vi "Get Tree Data for Affected Item.vi"(7 "Action":T2, 10 "User VI Ref":refnum<vi>, 11 "Affected Items":T3) -> (2 "Use Dialog?":bool, 3 "Elements Array":T1[](array[typedef]))   [LabVIEW 2023]
doc: "Given one of the affected items, return the associated cluster type of that item.\n\nIf action is Rearrange or Delete, this will be an array of strings of the unble or unbundle by name terminals."
uses:
  top/BundleMagic.ctl
  controls/action enum.ctl
  cluster/Cluster Element Description.ctl
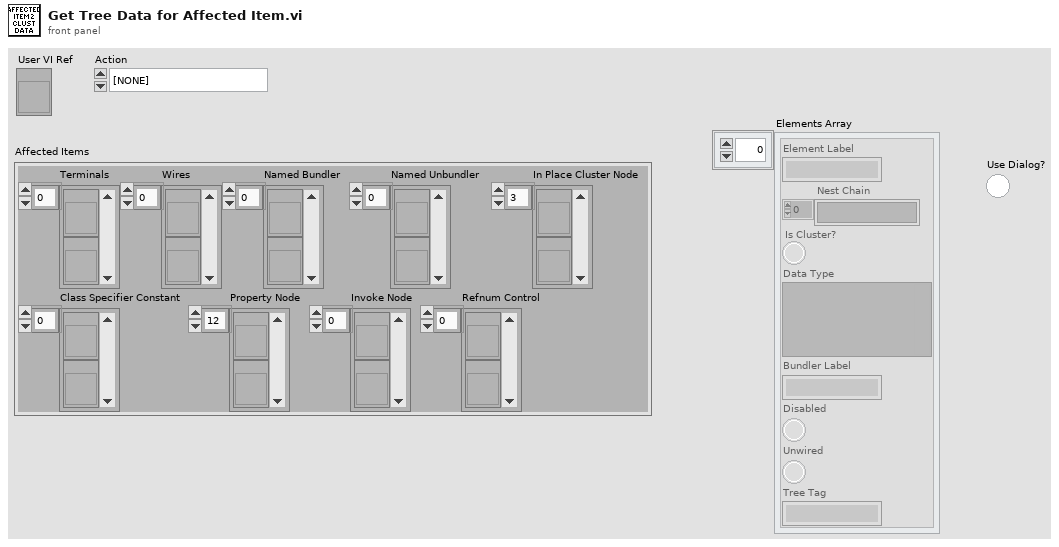
[diagram p1: front panel]
types:
  T1 = typedef "Cluster Element Description.ctl" = cluster{"Element Label":string, "Nest Chain":string[], "Is Cluster?":bool, "Data Type":variant, "Bundler Label":string, "Disabled":bool, "Unwired":bool, "Tree Tag":string}
  T2 = typedef "action enum.ctl" = enum16{"[NONE]", "Wire Bundle", "Wire Unbundle", "Terminal Unbundle", "Terminal Bundle", "Bundler Move Up", "Bundler Move Down", "Bundler Insert", "Bundler Remove", "Bundler Remove Unwired", "Bundler Rearrange", "In Place Insert", "In Place Remove", "In Place Remove Unwired", "In Place Rearrange", "Wire Properties", "Wire Method", "Terminal Properties", "Terminal Method", "Property Move Up", "Property Move Down", "Properties Insert", "Properties Remove", "Properties Remove Unwired", "Properties Rearrange", "Method Change", "Class for Constant", "Class For Control", "Class For Node", "Class Name to Clipboard"}
  T3 = typedef "BundleMagic.ctl" = cluster{"Terminals":refnum<vi>[], "Wires":refnum<vi>[], "Named Bundler":refnum<vi>[], "Named Unbundler":refnum<vi>[], "In Place Cluster Node":refnum<vi>[], "Class Specifier Constant":refnum<vi>[], "Property Node":refnum<vi>[], "Invoke Node":refnum<vi>[], "Refnum Control":refnum<vi>[]}
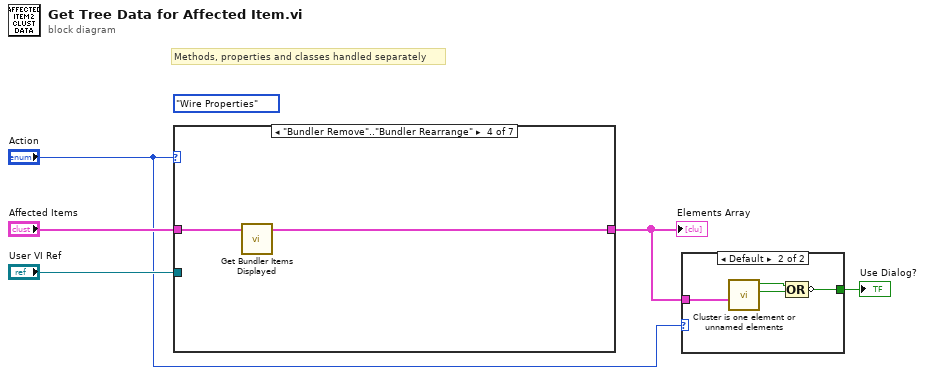
[diagram p0: block diagram]
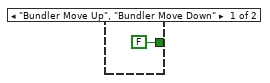
[diagram p2: hidden frame]
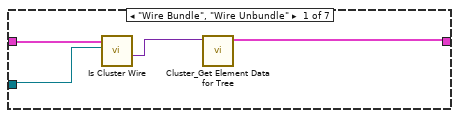
[diagram p3: hidden frame]
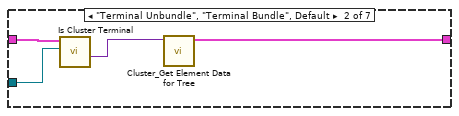
[diagram p4: hidden frame]
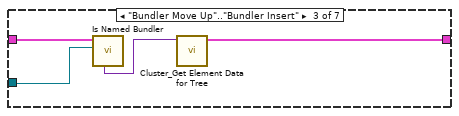
[diagram p5: hidden frame]
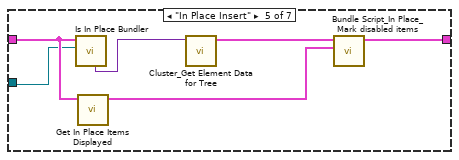
[diagram p6: hidden frame]
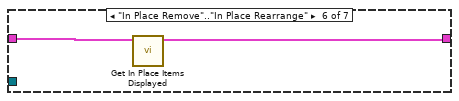
[diagram p7: hidden frame]
diagram:
  (unwired) action_enum."Wire Properties" ("Action")
  # "Methods, properties and classes handled separately"
  n1 = case shown="\"Bundler Remove\"..\"Bundler Rearrange\"" "Action" {
    tunnel: "Affected Items" -> [w9 w13 w17 w19 w24 w27 _]
    tunnel: "User VI Ref" -> [w8 w12 w16 _ w22 _ _]
    tunnel: [w6 w10 w14 w18 w23 w26 _] -> w2
    frame "Wire Bundle", "Wire Unbundle" {
      n2 = call "Is Cluster Wire.vi"("User VI Ref"=w8, "Affected Items"=w9) -> ("Data Type"=w7:variant)  [unwired: 6 in, 3 out]
      n3 = call "Cluster_Get Element Data for Tree.vi"("Data Type"=w7) -> ("Cluster Element Data Aray"=w6:T1[])  [unwired: 10 in]
    }
    frame "Terminal Unbundle", "Terminal Bundle", Default {
      n4 = call "Is Cluster Terminal.vi"("User VI Ref"=w12, "Affected Items"=w13) -> ("Data Type"=w11:variant)  [unwired: 7 in, 2 out]
      n5 = call "Cluster_Get Element Data for Tree.vi"("Data Type"=w11) -> ("Cluster Element Data Aray"=w10:T1[])  [unwired: 10 in]
    }
    frame "Bundler Move Up".."Bundler Insert" {
      n6 = call "Is Named Bundler.vi"("User VI Ref"=w16, "Affected Items"=w17) -> ("Data Type"=w15:variant)  [unwired: 3 in, 6 out]
      n7 = call "Cluster_Get Element Data for Tree.vi"("Data Type"=w15) -> ("Cluster Element Data Aray"=w14:T1[])  [unwired: 10 in]
    }
    frame "Bundler Remove".."Bundler Rearrange" {
      n8 = call "Get Bundler Items Displayed.vi"("Affected Items"=w19) -> ("Displayed Items"=w18:T1[])  [unwired: 10 in]
    }
    frame "In Place Insert" {
      n9 = call "Is In Place Bundler.vi"("User VI Ref"=w22, "Affected Items"=w24) -> ("Data Type"=w21:variant)  [unwired: 6 in, 3 out]
      n10 = call "Get In Place Items Displayed.vi"("Affected Items"=w24) -> ("Displayed Items"=w25:T1[])  [unwired: 10 in]
      n11 = call "Cluster_Get Element Data for Tree.vi"("Data Type"=w21) -> ("Cluster Element Data Aray"=w20:T1[])  [unwired: 10 in]
      n12 = call "Bundle Script_In Place_Mark disabled items.vi"("Displayed Items"=w25, "Cluster Items"=w20) -> ("Dialog Items"=w23:T1[])  [unwired: 9 in]
    }
    frame "In Place Remove".."In Place Rearrange" {
      n13 = call "Get In Place Items Displayed.vi"("Affected Items"=w27) -> ("Displayed Items"=w26:T1[])  [unwired: 10 in]
    }
    frame "[NONE]" {
    }
  }
  "Elements Array" <- w2
  n14 = case shown="Default" "Action" {
    tunnel: [FALSE w30] -> w3
    tunnel: w2 -> [_ w29]
    frame "Bundler Move Up", "Bundler Move Down" {
    }
    frame Default {
      n15 = call "Cluster is one element or unnamed elements.vi"("Cluster Elements Array"=w29) -> ("All Unnamed?"=w31:bool, "One Element?"=w32:bool)  [unwired: 8 in, 1 out]
      n16 = Compound Arithmetic op=OR(w32, w31) -> (invert w30:bool)
    }
  }
  "Use Dialog?" <- w3
